vi "软边光阑2.vi"(5 "error in (no error)":errorcluster) -> (0 "error out":errorcluster, 1 "CH2":dbl[][](array[numeric]), 2 "CH1":dbl[][](array[numeric]))   [LabVIEW 2018]
uses:
  LeCroy Wave Series/Public/Configure/Configure Edge Trigger.vi
  LeCroy Wave Series/Public/Data/Read Multiple Waveforms.vi
  LeCroy Wave Series/LeCroy Wave Series.lvlib
panel:
  out "大小":i32
  out "CH2":waveform(dbl)(graph)
  out "code":i32
  out "CH3":waveform(dbl)(graph)
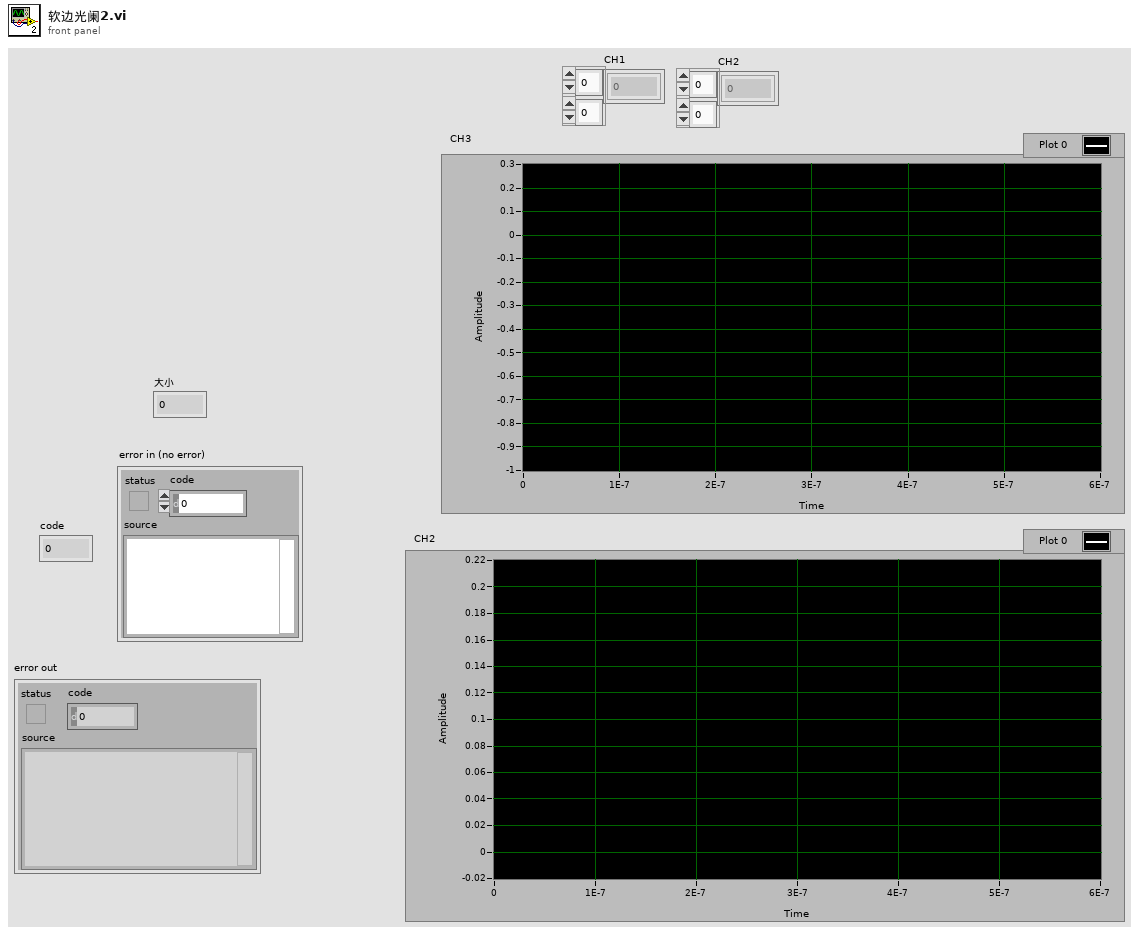
[diagram p1: front panel]
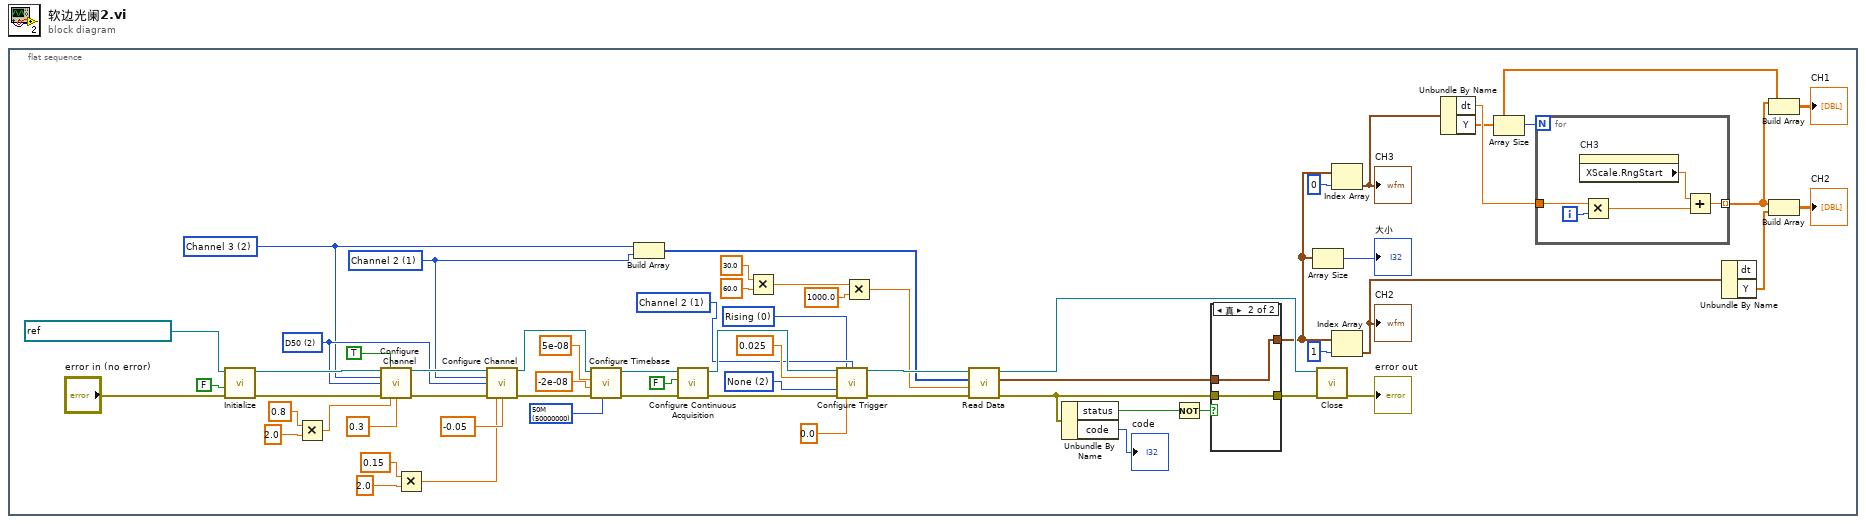
[diagram p0: block diagram]
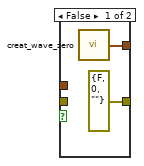
[diagram p2: hidden frame]
diagram:
  n1 = flat-sequence {
    frame #0 {
      w18 = u16 1 items=["Channel 1", "Channel 2", "Channel 3", "Channel 4"] ("Channel (0: Channel 1)")
      w22 = u16 2 items=["Channel 1", "Channel 2", "Channel 3", "Channel 4"] ("Channel (0: Channel 1)")
      w53 = 50000000 items=["50"=50, "100"=100, "250"=250, "500"=500, "1000"=1000, "2500"=2500, "5K"=5000, "10K"=10000, "25K"=25000, "50K"=50000, "100K"=100000, "250K"=250000, "500K"=500000, "1M"=1000000, "2M"=2000000, "2.5M"=2500000, "5M"=5000000, "10M"=10000000, "25M"=25000000, "50M"=50000000, "100M"=100000000] ("Maximum Sample Points (500)")
      w27 = u16 2 items=["A1M", "D1M", "D50", "Ground", "DC", "AC"] ("Vertical Coupling (0: A1M)")
      w50 = u16 1 items=["Channel 1", "Channel 2", "Channel 3", "Channel 4", "External", "Line", "Ext", "Ext10"] ("Trigger Source (0: Channel 1)")
      w49 = u16 0 items=["Rising", "Falling"] ("Trigger Slope (0: Rising)")
      w44 = u16 2 items=["Time", "Events", "None"] ("Holdoff Type (0: Time)")
      n2 = call "Initialize.vi"("error in (no error)"="error in (no error)", "Reset? (T: Yes)"=FALSE, "VISA resource name"=refnum<visa-resource-name> "VICP::192.168.129.96") -> ("error out"=w58:errorcluster, "VISA resource name out"=w61:refnum<visa-resource-name>)  [unwired: 7 in]
      n3 = Multiply(x=0.8, y=2.0) -> (x*y=w47:dbl)
      n4 = call "Configure Channel.vi"("VISA resource name"=w61, "Enable Channel (T:On)"=TRUE, "Channel (0: Channel 1)"=w22, "Vertical Coupling (0: A1M)"=w27, "error in (no error)"=w58, "Vertical Range (10.0 V)"=w47, "Vertical Offset (0.0 V)"=0.3) -> ("VISA resource name out"=w31:refnum<visa-resource-name>, "error out"=w29:errorcluster)  [unwired: 7 in]
      n5 = Multiply(x=0.15, y=2.0) -> (x*y=w23:dbl)
      n6 = call "Configure Channel.vi"("VISA resource name"=w31, "Channel (0: Channel 1)"=w18, "Vertical Coupling (0: A1M)"=w27, "error in (no error)"=w29, "Vertical Range (10.0 V)"=w23, "Vertical Offset (0.0 V)"=-0.05) -> ("VISA resource name out"=w30:refnum<visa-resource-name>, "error out"=w28:errorcluster)  [unwired: 8 in]
      n7 = call "Configure Timebase.vi"("Maximum Sample Points (500)"=w53, "error in (no error)"=w28, "Position (0.0 s)"=-2e-08, "Timebase (0.0005 s)"=5e-08, "VISA resource name"=w30) -> ("error out"=w57:errorcluster, "VISA resource name out"=w60:refnum<visa-resource-name>)  [unwired: 5 in]
      n8 = Build Array(w22, w18) -> (w21:u16[])
      n9 = call "Configure Continuous Acquisition.vi"("error in (no error)"=w57, "Continuous Acquisition Mode (T: On)"=FALSE, "VISA resource name"=w60) -> ("error out"=w56:errorcluster, "VISA resource name out"=w59:refnum<visa-resource-name>)  [unwired: 7 in]
      n10 = Multiply(x=30.0, y=60.0) -> (x*y=w36:dbl)
      n11 = call-poly "Configure Trigger.vi"("VISA resource name"=w59, "Trigger Slope (0: Rising)"=w49, "Trigger Source (0: Channel 1)"=w50, "Trigger Level (0.0 V)"=0.025, "Holdoff Type (0: Time)"=w44, "error in (no error)"=w56, "Holdoff Value by Time (50 ns)"=0.0) -> ("VISA resource name out"=w43:refnum<visa-resource-name>, "error out"=w42:errorcluster)  [unwired: 7 in]
      n12 = Multiply(x=w36, y=1000.0) -> (x*y=w32:dbl)
      n13 = call-poly "Read Data.vi"("error in (no error)"=w42, "Timeout (10000 ms)"=w32, "Channels"=w21, "VISA resource name"=w43) -> ("error out"=w5:errorcluster, "Waveform Data"=w4:waveform(dbl)[], "VISA resource name out"=w41:refnum<visa-resource-name>)  [unwired: 5 in]
      n14 = Unbundle By Name(w5) -> ("status"=w38:bool, "code"=→"code":i32)
      n15 = Not(x=w38) -> (.not. x?=w2:bool)
      n16 = case shown="真" w2 {
        tunnel: [w70 w71] -> w3
        tunnel: [errorcluster {"status"=FALSE, "code"=0, "source"=""} ("error in (no error) 2") w72] -> w1
        tunnel: w5 -> [_ w72]
        tunnel: w4 -> [_ w71]
        frame False {
          n17 = call "creat_wave_zero.vi"() -> ("添加的数组"=w70:waveform(dbl)[])  [unwired: 1 in]
        }
        frame True {
        }
      }
      n18 = Array Size(array=w3) -> (size(s)=→"大小":i32)
      n19 = call "Close.vi"("error in (no error)"=w1, "VISA resource name"=w41) -> ("error out"=→"error out":errorcluster)  [unwired: 9 in]
      n20 = Index Array(array=w3, index=0 ("索引")) -> (element=w11:waveform(dbl))
      "CH3" <- w11
      n21 = Index Array(array=w3, index=1 ("索引")) -> (element=w15:waveform(dbl))
      "CH2" <- w15
      n22 = Unbundle By Name(w11) -> ("dt"=w13:dbl, "Y"=w6:dbl[])
      n23 = Array Size(array=w6) -> (size(s)=w12:i32)
      n24 = for {
        N: w12 -> [_]
        tunnel: [w67] -> w9 mode=indexing
        tunnel: w13 -> [w64]
        i -> [w66]
        n25 = property on="CH3" class="WFGraph (严格)"() -> ("XScale.RngStart"=w68:dbl)  [unwired: 2 in, 2 out]
        n26 = Multiply(x=w64, y=w66) -> (x*y=w65:dbl)
        n27 = Add(x=w68, y=w65) -> (x+y=w67:dbl)
      }
      n28 = Unbundle By Name(w15) -> ("Y"=w10:dbl[])  [unwired: 1 out]
      n29 = Build Array(w9, w6) -> (→"CH1":dbl[][])
      n30 = Build Array(w9, w10) -> (→"CH2":dbl[][])
    }
  }
